vi "DAQ_OPC UA.vi"() -> (0 "Error Out":errorcluster)   [LabVIEW 2017]
uses:
  <vilib>/dex/Flush And Wait Empty Condition.ctl
  <vilib>/Platform/TimedLoop/XDataNode/timing_clust.ctl
  <vilib>/Platform/TimedLoop/XDataNode/nitl_modes.ctl
  <vilib>/Platform/TimedLoop/XDataNode/wakeup.ctl
  <vilib>/DAQmx/read.llb/DAQmx Read (Analog 1D DBL NChan 1Samp).vi
  <vilib>/DAQmx/miscellaneous.llb/DAQmx Fill In Error Info.vi
  <vilib>/Platform/TimedLoop/XDataNode/XDataNode.xnode
  <vilib>/Platform/TimedLoop/XDataNode/XDNodeRunTimeDep.lvlib
  <resource>/objmgr/ni.dex.rc
panel:
  out "Producer Loop Time":i64
  out "Consumer Loop Time":u32
  out "Time":dbl
  out "Available Elements for Writing":i32
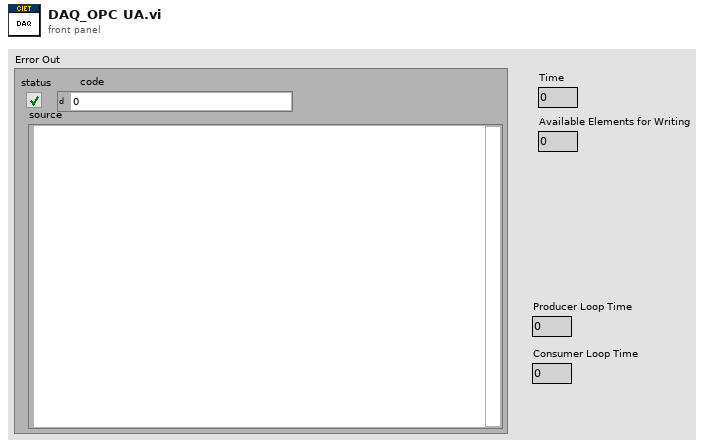
[diagram p1: front panel]
types:
  T1 = typedef "Flush And Wait Empty Condition.ctl" = u8
  T2 = typedef "XDNodeRunTimeDep.lvlib/timing_clust.ctl" = cluster{"Expected End [f-1]":u64, "Actual End [f-1]":u64, "Finished Late? [f-1]":bool, "Expected End [i-1]":u64, "Actual End [i-1]":u64, "Finished Late? [i-1]":bool, "Expected Start [i]":u64, "Actual Start [i]":u64, "Expected Start [f]":u64, "Actual Start [f]":u64, "Source Name":string, "Structure Name":string, "Period":i64, "Deadline":i64, "Offset":i64, "Start":i64, "Priority":i32, "Timeout":i32, "Mode":T3, "Wakeup Reason":T4, "Error":errorcluster, "Source Type":string, "Secondary Source Type":string, "Global End Time":u64, "Global Start Time":u64, "Frame Duration":u64, "Iteration Duration":u64, "Assigned CPU":i32, "I/O Scan Engine Mode":u32}
  T3 = typedef "XDNodeRunTimeDep.lvlib/nitl_modes.ctl" = enum32{"No Change", "Process missed periods, maintain original phase", "Discard missed periods, maintain original phase", "Process missed periods, ignore original phase", "Discard missed periods, ignore original phase"}
  T4 = typedef "XDNodeRunTimeDep.lvlib/wakeup.ctl" = enum32{"Normal", "Aborted", "Asynchronous wakeup", "Timing source error", "Timed loop error", "Timeout"}
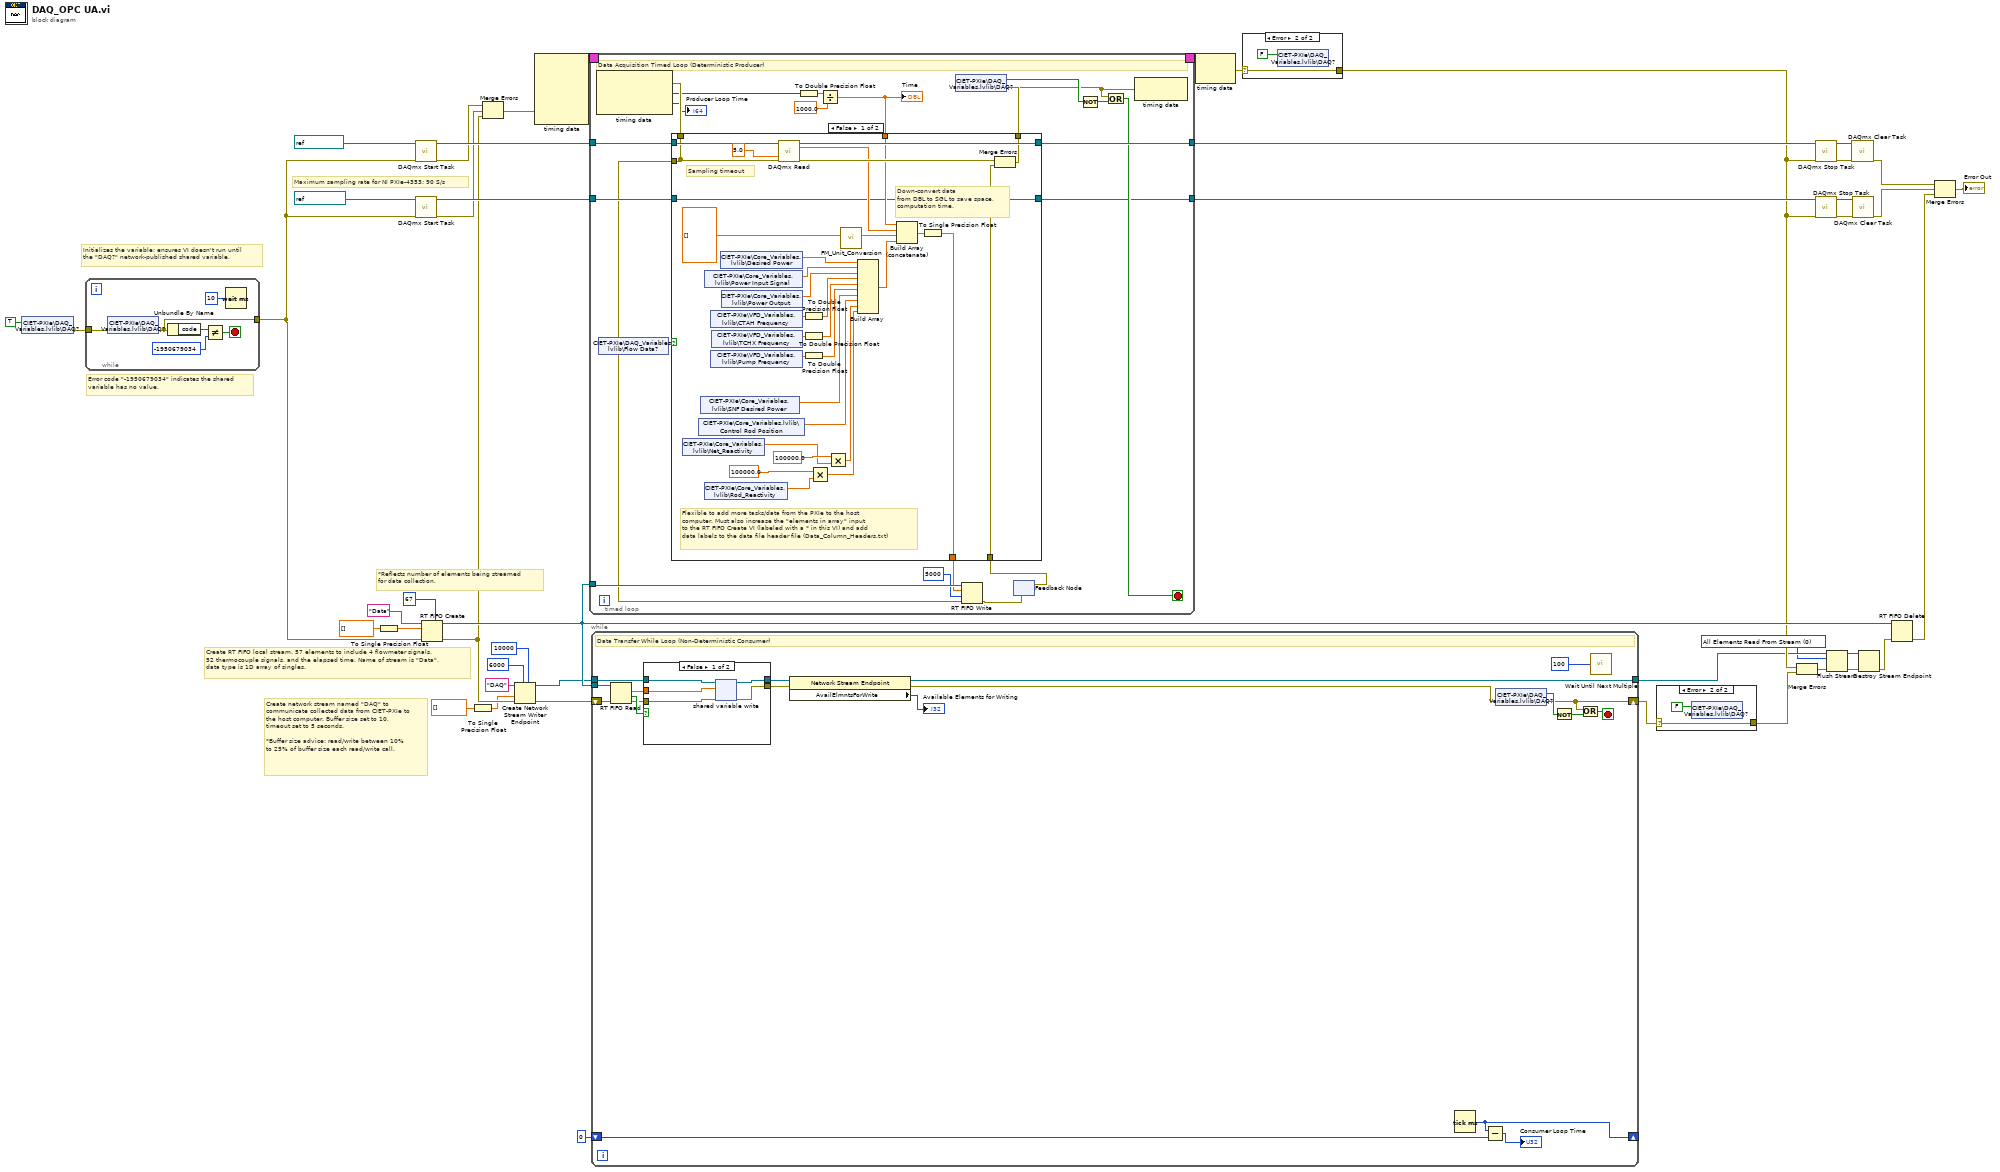
[diagram p0: block diagram]
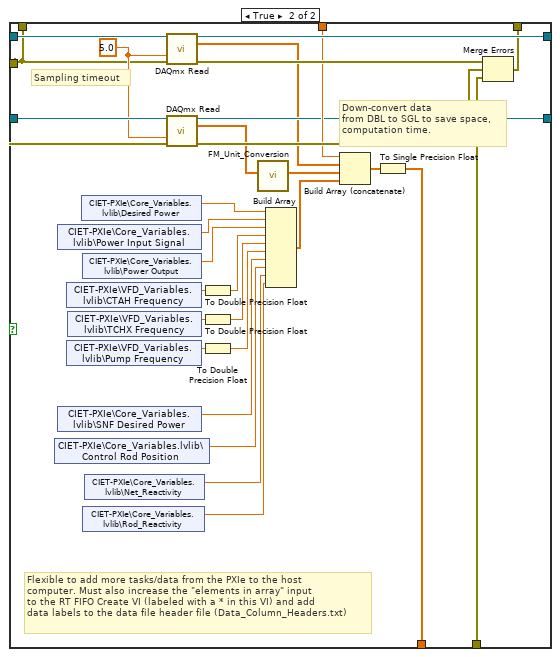
[diagram p5: hidden frame]
diagram:
  w2 = T1 0 items=["All Elements Read From Stream", "All Elements Available for Reading"] ("wait condition")
  # "*Reflects number of elements being streamed\nfor data collection."
  # "Create RT FIFO local stream. 57 elements to include 4 flowmeter signals,\n52 thermocouple signals, and the elapsed time. Name of stream is \"Data\",\ndata type is 1D array of singles."
  # "Create network stream named \"DAQ\" to communicate collected data from CIET-PXIe to the host computer. Buffer size set to 10, timeout set to 5 seconds. \n\n*Buffer size advice: read/write between 10%\nto 25% of buffer size each read/write call."
  # "Maximum sampling rate for NI PXIe-4353: 90 S/s"
  # "Initializes the variable; ensures VI doesn't run until\nthe \"DAQ?\" network-published shared variable."
  # "Error code \"-1950679034\" indicates the shared\nvariable has no value."
  n1 = shared-variable "CIET-PXIe\\DAQ_Variables.lvlib\\DAQ?"(TRUE ("Active?")) -> (error out=w22:errorcluster)  [unwired: 1 in]
  n2 = while {
    tunnel: w22 -> [w51]
    tunnel: [w50] -> w21
    stop <- w47 stop-if-true
    n3 = shared-variable "CIET-PXIe\\DAQ_Variables.lvlib\\DAQ?"(error in=w51) -> (error out=w50:errorcluster)  [unwired: 1 out]
    n4 = Unbundle By Name(w50) -> ("code"=w49:i32)
    n5 = Not Equal?(x=w49, y=-1950679034) -> (x != y?=w47:bool)
    n6 = Wait (ms)(milliseconds to wait=u32 10) -> ()  [unwired: 1 out]
  }
  n7 = To Single Precision Float(number=dbl[] []) -> (single precision float=w32:sgl[])
  n8 = call <vilib>:"DAQmx Start Task.vi"("task/channels in"=refnum<k21> "CIET-TC", "error in"=w21) -> ("task out"=w42:refnum<k21>, "error out"=w26:errorcluster)  [unwired: 12 in]
  n9 = call <vilib>:"DAQmx Start Task.vi"("task/channels in"=refnum<k21> "CIET-FM", "error in"=w21) -> ("task out"=w41:refnum<k21>, "error out"=w27:errorcluster)  [unwired: 12 in]
  n10 = RT FIFO Create(0:"Data" ("name (unnamed)"), 1:w32, 3:w21, 6:u32 67 ("elements in array (1)")) -> (8:w25:refnum<k33>, 11:w17:errorcluster)  [unwired: 4 in, 1 out]
  n11 = To Single Precision Float(number=dbl[] []) -> (single precision float=w7:sgl[])
  n12 = Merge Errors(w26, w27, w17) -> (w28:errorcluster)
  n13 = Create Network Stream Writer Endpoint(5:10000 ("timeout in ms (-1)"), 7:6000 ("writer buffer size"), 8:w17, 9:w7, 11:"DAQ" ("writer name")) -> (0:w18:errorcluster, 3:w16:refnum<k21>)  [unwired: 2 in]
  n14 = node-c288(w28) -> (w46:T2)  [unwired: 4 in]
  n15 = timed-loop {
    timing: w46 -> [_]
    timing-out: [_] -> w45
    tunnel: w25 -> [w71]
    tunnel: w42 -> [w74]
    tunnel: [w72] -> w36
    tunnel: w41 -> [w73]
    tunnel: [w59] -> w35
    stop <- w66 stop-if-true
    # "Data Acquisition Timed Loop (Deterministic Producer)"
    n16 = node-c288() -> (w69:errorcluster, w60:i64, →"Producer Loop Time":i64)  [unwired: 1 in]
    n17 = shared-variable "CIET-PXIe\\DAQ_Variables.lvlib\\Flow Data?"() -> (w54:bool)  [unwired: 1 in, 1 out]
    n18 = To Double Precision Float(number=w60) -> (double precision float=w63:dbl)
    n19 = Divide(x=w63, y=1000.0) -> (x/y=w62:dbl)
    "Time" <- w62
    n20 = feedback #1() -> (w55:errorcluster)  [unwired: 1 in]
    n21 = case shown="False" w54 {
      tunnel: w74 -> [w106 w136]
      tunnel: w73 -> [w86 w135]
      tunnel: [w104 w133] -> w72
      tunnel: [w102 w131] -> w57
      tunnel: w69 -> [w83 w111]
      tunnel: w55 -> [w84 w128]
      tunnel: [w100 w127] -> w65
      tunnel: w62 -> [w99 w126]
      tunnel: [w86 w125] -> w59
      tunnel: [w83 w111] -> w53
      frame False {
        # "Flexible to add more tasks/data from the PXIe to the host \ncomputer. Must also increase the \"elements in array\" input \nto the RT FIFO Create VI (labeled with a * in this VI) and add\ndata labels to the data file header file (Data_Column_Headers.txt)"
        # "Down-convert data\nfrom DBL to SGL to save space,\ncomputation time."
        # "Sampling timeout"
        n22 = shared-variable "CIET-PXIe\\Core_Variables.lvlib\\Net_Reactivity"() -> (w76:dbl)  [unwired: 1 in, 1 out]
        n23 = shared-variable "CIET-PXIe\\Core_Variables.lvlib\\Control Rod Position"() -> (w81:dbl)  [unwired: 1 in, 1 out]
        n24 = shared-variable "CIET-PXIe\\Core_Variables.lvlib\\SNF Desired Power"() -> (w82:dbl)  [unwired: 1 in, 1 out]
        n25 = shared-variable "CIET-PXIe\\Core_Variables.lvlib\\Power Input Signal"() -> (w89:dbl)  [unwired: 1 in, 1 out]
        n26 = shared-variable "CIET-PXIe\\Core_Variables.lvlib\\Rod_Reactivity"() -> (w79:dbl)  [unwired: 1 in, 1 out]
        n27 = shared-variable "CIET-PXIe\\VFD_Variables.lvlib\\CTAH Frequency"() -> (w91:sgl)  [unwired: 1 in, 1 out]
        n28 = shared-variable "CIET-PXIe\\VFD_Variables.lvlib\\Pump Frequency"() -> (w93:sgl)  [unwired: 1 in, 1 out]
        n29 = shared-variable "CIET-PXIe\\VFD_Variables.lvlib\\TCHX Frequency"() -> (w92:sgl)  [unwired: 1 in, 1 out]
        n30 = shared-variable "CIET-PXIe\\Core_Variables.lvlib\\Desired Power"() -> (w88:dbl)  [unwired: 1 in, 1 out]
        n31 = shared-variable "CIET-PXIe\\Core_Variables.lvlib\\Power Output"() -> (w90:dbl)  [unwired: 1 in, 1 out]
        n32 = call-poly <vilib>:"DAQmx Read.vi"("task/channels in"=w106, "timeout"=5.0, "error in"=w83) -> ("task out"=w104:refnum<k21>, "data"=w98:dbl[], "error out"=w101:errorcluster)  [unwired: 10 in]
        n33 = To Double Precision Float(number=w91) -> (double precision float=w94:dbl)
        n34 = To Double Precision Float(number=w92) -> (double precision float=w95:dbl)
        n35 = To Double Precision Float(number=w93) -> (double precision float=w96:dbl)
        n36 = Multiply(x=100000.0 ("y"), y=w79) -> (x*y=w78:dbl)
        n37 = Multiply(x=100000.0 ("y"), y=w76) -> (x*y=w75:dbl)
        n38 = call "FM_Unit_Conversion.vi"("Input Array [A]"=dbl[] []) -> ("Output Array [kg/h]"=w97:dbl[])  [unwired: 10 in]
        n39 = Build Array(w88, w89, w90, w94, w95, w96, w82, w81, w75, w78) -> (w87:dbl[])
        n40 = Build Array (concatenate)(w99, w98, w97, w87) -> (w103:dbl[])
        n41 = To Single Precision Float(number=w103) -> (single precision float=w102:sgl[])
        n42 = Merge Errors(w101, w84) -> (w100:errorcluster)
      }
      frame True {
        w134 = 5.0 ("timeout")
        # "Flexible to add more tasks/data from the PXIe to the host \ncomputer. Must also increase the \"elements in array\" input \nto the RT FIFO Create VI (labeled with a * in this VI) and add\ndata labels to the data file header file (Data_Column_Headers.txt)"
        # "Down-convert data\nfrom DBL to SGL to save space,\ncomputation time."
        # "Sampling timeout"
        n43 = shared-variable "CIET-PXIe\\Core_Variables.lvlib\\Control Rod Position"() -> (w109:dbl)  [unwired: 1 in, 1 out]
        n44 = shared-variable "CIET-PXIe\\Core_Variables.lvlib\\Power Input Signal"() -> (w114:dbl)  [unwired: 1 in, 1 out]
        n45 = shared-variable "CIET-PXIe\\Core_Variables.lvlib\\SNF Desired Power"() -> (w110:dbl)  [unwired: 1 in, 1 out]
        n46 = shared-variable "CIET-PXIe\\VFD_Variables.lvlib\\CTAH Frequency"() -> (w116:sgl)  [unwired: 1 in, 1 out]
        n47 = shared-variable "CIET-PXIe\\VFD_Variables.lvlib\\Pump Frequency"() -> (w118:sgl)  [unwired: 1 in, 1 out]
        n48 = shared-variable "CIET-PXIe\\VFD_Variables.lvlib\\TCHX Frequency"() -> (w117:sgl)  [unwired: 1 in, 1 out]
        n49 = shared-variable "CIET-PXIe\\Core_Variables.lvlib\\Desired Power"() -> (w113:dbl)  [unwired: 1 in, 1 out]
        n50 = shared-variable "CIET-PXIe\\Core_Variables.lvlib\\Power Output"() -> (w115:dbl)  [unwired: 1 in, 1 out]
        n51 = shared-variable "CIET-PXIe\\Core_Variables.lvlib\\Rod_Reactivity"() -> (w107:dbl)  [unwired: 1 in, 1 out]
        n52 = shared-variable "CIET-PXIe\\Core_Variables.lvlib\\Net_Reactivity"() -> (w108:dbl)  [unwired: 1 in, 1 out]
        n53 = call-poly <vilib>:"DAQmx Read.vi"("task/channels in"=w136, "timeout"=w134, "error in"=w111) -> ("task out"=w133:refnum<k21>, "data"=w124:dbl[], "error out"=w129:errorcluster)  [unwired: 10 in]
        n54 = call-poly <vilib>:"DAQmx Read.vi"("task/channels in"=w135, "timeout"=w134, "error in"=w111) -> ("task out"=w125:refnum<k21>, "data"=w122:dbl[], "error out"=w130:errorcluster)  [unwired: 10 in]
        n55 = To Double Precision Float(number=w116) -> (double precision float=w119:dbl)
        n56 = To Double Precision Float(number=w117) -> (double precision float=w120:dbl)
        n57 = To Double Precision Float(number=w118) -> (double precision float=w121:dbl)
        n58 = call "FM_Unit_Conversion.vi"("Input Array [A]"=w122) -> ("Output Array [kg/h]"=w123:dbl[])  [unwired: 10 in]
        n59 = Build Array(w113, w114, w115, w119, w120, w121, w110, w109, w108, w107) -> (w112:dbl[])
        n60 = Build Array (concatenate)(w126, w124, w123, w112) -> (w132:dbl[])
        n61 = To Single Precision Float(number=w132) -> (single precision float=w131:sgl[])
        n62 = Merge Errors(w129, w130, w128) -> (w127:errorcluster)
      }
    }
    n63 = shared-variable "CIET-PXIe\\DAQ_Variables.lvlib\\DAQ?"(error in=w65) -> (w68:bool, error out=w64:errorcluster)
    n64 = RT FIFO Write(0:w71, 1:w57, 2:5000 ("timeout in ms (0)"), 3:w53) -> (11:w56:errorcluster)  [unwired: 1 in, 3 out]
    n65 = feedback-in #1(w56) -> ()
    n66 = Not(x=w68) -> (.not. x?=w67:bool)
    n67 = Or(x=w64, y=w67) -> (x .or. y?=w66:bool)
    n68 = node-c288(w64) -> ()  [unwired: 1 out]
  }
  n69 = while {
    tunnel: w25 -> [w162]
    shift-right: [w151] -> w19
    shift-left: w18 -> [w161]
    tunnel: w16 -> [w153]
    tunnel: [w148] -> w9
    shift-right: [w146] -> _
    shift-left: u32 0 ("millisecond timer value") -> [w145]
    stop <- w154 stop-if-true
    # "Data Transfer While Loop (Non-Deterministic Consumer)"
    n70 = RT FIFO Read(0:w162, 3:w161) -> (9:w158:sgl[], 10:w159:bool, 11:w157:errorcluster)  [unwired: 2 in, 2 out]
    n71 = case shown="False" w159 {
      tunnel: w158 -> [w163 _]
      tunnel: w157 -> [w167 w169]
      tunnel: [w166 w169] -> w150
      tunnel: w153 -> [w165 w168]
      tunnel: [w164 w168] -> w149
      frame False {
        n72 = shared-variable-write(w165, w167, w163) -> (w164:refnum<k21>, w166:errorcluster)  [unwired: 1 in, 1 out]
      }
      frame True {
      }
    }
    n73 = property class="Network Stream Endpoint"(reference=w149, error in=w150) -> (reference out=w148:refnum<k21>, error out=w147:errorcluster, "AvailElmntsForWrite"=→"Available Elements for Writing":i32)
    n74 = Tick Count (ms)() -> (millisecond timer value=w146:u32)
    n75 = Subtract(x=w146, y=w145) -> (x-y=→"Consumer Loop Time":u32)
    n76 = shared-variable "CIET-PXIe\\DAQ_Variables.lvlib\\DAQ?"(error in=w147) -> (w156:bool, error out=w151:errorcluster)
    n77 = Not(x=w156) -> (.not. x?=w155:bool)
    n78 = Or(x=w151, y=w155) -> (x .or. y?=w154:bool)
    n79 = call "Wait Until Next Multiple"("Count(mSec)"=u32 100) -> ()  [unwired: 1 out]
  }
  n80 = node-c288(w45) -> (w20:errorcluster)
  n81 = case shown="Error" w20 {
    selector: w20 -> [w170 w171]
    tunnel: [w170 w171] -> w15
    frame No Error {
    }
    frame Error {
      n82 = shared-variable "CIET-PXIe\\DAQ_Variables.lvlib\\DAQ?"(FALSE ("DAQ?")) -> ()  [unwired: 1 in, 1 out]
    }
  }
  n83 = case shown="Error" w19 {
    selector: w19 -> [w173 w174]
    tunnel: [w173 w174] -> w14
    frame No Error {
    }
    frame Error {
      n84 = shared-variable "CIET-PXIe\\DAQ_Variables.lvlib\\DAQ?"(FALSE ("DAQ?")) -> ()  [unwired: 1 in, 1 out]
    }
  }
  n85 = Merge Errors(w15, w14) -> (w11:errorcluster)
  n86 = call <vilib>:"DAQmx Stop Task.vi"("task/channels in"=w36, "error in"=w15) -> ("task out"=w39:refnum<k21>, "error out"=w40:errorcluster)  [unwired: 12 in]
  n87 = call <vilib>:"DAQmx Stop Task.vi"("task/channels in"=w35, "error in"=w15) -> ("task out"=w37:refnum<k21>, "error out"=w38:errorcluster)  [unwired: 12 in]
  n88 = Flush Stream(8:w11, 10:w2, 11:w9) -> (0:w13:errorcluster, 3:w12:refnum<k21>)  [unwired: 1 in, 1 out]
  n89 = call <vilib>:"DAQmx Clear Task.vi"("task in"=w39, "error in"=w40) -> ("error out"=w34:errorcluster)  [unwired: 13 in]
  n90 = call <vilib>:"DAQmx Clear Task.vi"("task in"=w37, "error in"=w38) -> ("error out"=w33:errorcluster)  [unwired: 13 in]
  n91 = Destroy Stream Endpoint(8:w13, 11:w12) -> (0:w10:errorcluster)
  n92 = RT FIFO Delete(0:w25, 3:w10) -> (11:w4:errorcluster)  [unwired: 1 in]
  n93 = Merge Errors(w34, w33, w4) -> (→"Error Out":errorcluster)
